vi "PH_OceanOpticsSpectrometer.SpectroAnalysis.vi"(0 "Spectrum":cluster{sgl[], "Master Data":sgl[]}, 1 "lower Limit":dbl=900.0, 2 "upper Limit":dbl=1000.0, 5 "error in (no error)":errorcluster) -> (14 "width":dbl format="%.2p", 15 "center wavelength":sgl, 19 "error out":errorcluster)   [LabVIEW 2014, in "PH_OceanOpticsSpectrometer.lvlib"]
uses:
  PH_OceanOpticsSpectrometer.lvlib
  <vilib>/measure/mascope.llb/Transition Measurements 1 chan (obs).vi
  <vilib>/measure/NI_MAPro.lvlib
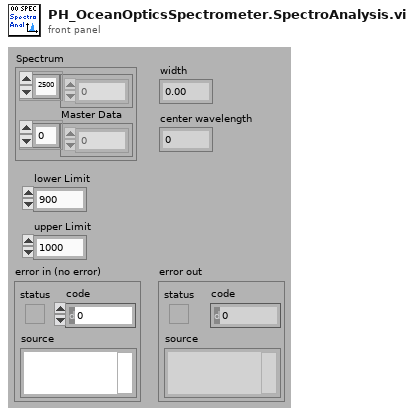
[diagram p1: front panel]
types:
  T1 = cluster{"high ref level":dbl, "mid ref level":dbl, "low ref level":dbl, "ref units":u16}
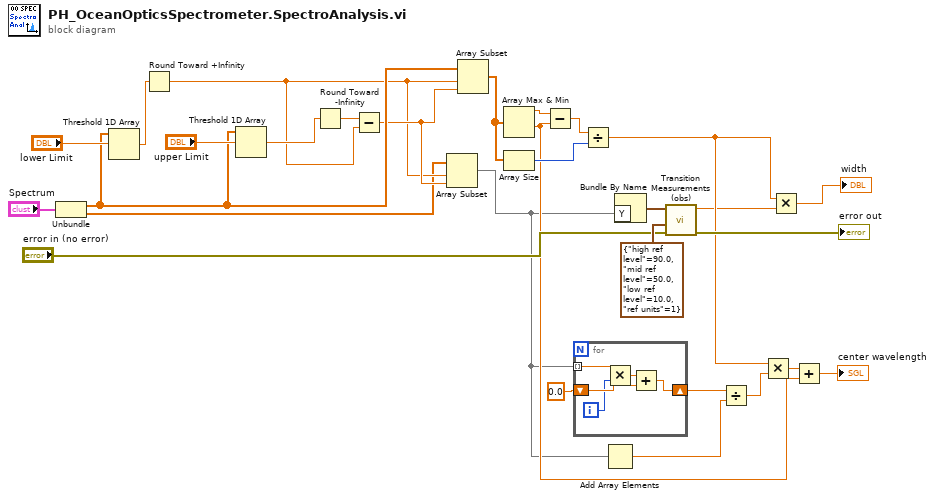
[diagram p0: block diagram]
diagram:
  n1 = Unbundle("Spectrum") -> (w6:sgl[], "Master Data"=w2:sgl[])
  n2 = Threshold 1D Array(2:"lower Limit", 3:w6) -> (0:w9:sgl)  [unwired: 1 in]
  n3 = Round Toward +Infinity(x=w9) -> (ceil(x): smallest int >= x=w3:sgl)
  n4 = Threshold 1D Array(2:"upper Limit", 3:w6) -> (0:w8:sgl)  [unwired: 1 in]
  n5 = Round Toward -Infinity(1:w8) -> (0:w7:sgl)
  n6 = Subtract(x=w7, y=w3) -> (x-y=w4:sgl)
  n7 = Array Subset(array=w2, index=w3, length=w4) -> (w1:sgl[])
  n8 = Array Subset(array=w6, index=w3, length=w4) -> (w5:sgl[])
  n9 = Array Max & Min(array=w5) -> (max value=w24:sgl, min value=w12:sgl)  [unwired: 2 out]
  n10 = Array Size(array=w5) -> (size(s)=w22:i32)
  n11 = Subtract(x=w24, y=w12) -> (x-y=w23:sgl)
  n12 = for {
    tunnel: w1 -> [w33] mode=indexing
    shift-right: [w34] -> w25
    shift-left: sgl 0.0 -> [w31]
    i -> [w30]
    n13 = Multiply(x=w33, y=w30) -> (x*y=w32:sgl)
    n14 = Add(x=w32, y=w31) -> (x+y=w34:sgl)
  }
  n15 = Divide(x=w23, y=w22) -> (x/y=w17:sgl)
  n16 = Add Array Elements(numeric array=w1) -> (sum=w14:sgl)
  n17 = Bundle By Name("Y"=w1) -> (w15:waveform(sgl))  [unwired: 1 in]
  n18 = call-poly <vilib>:"Transition Measurements (obs).vi"("error in (no error)"="error in (no error)", "reference levels"=T1 {"high ref level"=90.0, "mid ref level"=50.0, "low ref level"=10.0, "ref units"=1}, "signal in"=w15) -> ("error out"=→"error out":errorcluster, "duration"=w16:dbl)  [unwired: 3 in, 4 out]
  n19 = Divide(x=w25, y=w14) -> (x/y=w21:sgl)
  n20 = Multiply(x=w17, y=w21) -> (x*y=w19:sgl)
  n21 = Multiply(x=w17, y=w16) -> (x*y=→"width":dbl)
  n22 = Add(x=w19, y=w12) -> (x+y=→"center wavelength":sgl)
